vi "GET STOP.vi"(9 "error in (no error)":errorcluster) -> (8 "Boolean":bool, 10 "error out":errorcluster)   [LabVIEW 2013, in "GlobalStop(dev).lvlib"]
uses:
  GlobalStop(dev).lvlib
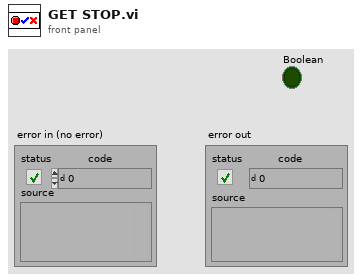
[diagram p1: front panel]
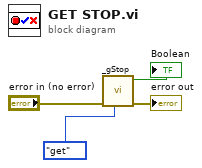
[diagram p0: block diagram]
diagram:
  n1 = call "_gStop.vi"("op"=enum16{"reset", "get", "stop"}."get", "error in (no error)"="error in (no error)") -> ("error out"=→"error out":errorcluster, "Boolean"=→"Boolean":bool)  [unwired: 8 in]
